vi "NI VeriStand - Get Custom Device Channel Value Table.vi"(8 "error in (no error)":errorcluster, 11 "Channel Ref in":T1 format="%.0x") -> (0 "error out":errorcluster, 1 "Values":dbl[](array[numeric]), 2 "Names":string[](array[string]), 3 "Channel Ref out":T1=18446744073709551615 format="%.0x")   [LabVIEW 2020, in "Custom Device API.lvlib"]
uses:
  <vilib>/NI VeriStand/Custom Device API/Custom Device API.lvlib
  <vilib>/NI VeriStand/Custom Device API/Custom Device Item Ref.ctl
  46f13d71-0576-4d04-b334-0d328d6cd7fa.vi
  <vilib>/NI VeriStand/Custom Device API/Custom Device Offline Path.vi
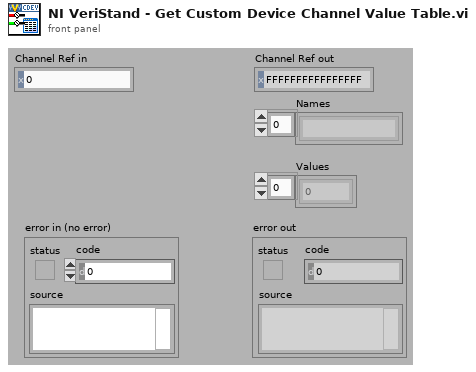
[diagram p1: front panel]
types:
  T1 = typedef "Custom Device API.lvlib/Custom Device Item Ref.ctl" = u64
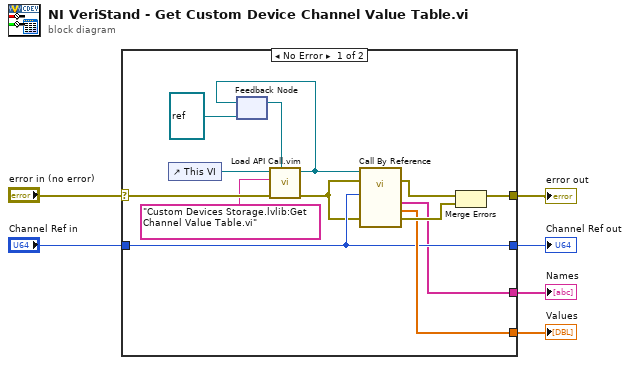
[diagram p0: block diagram]
diagram:
  n1 = case shown="No Error" "error in (no error)" {
    selector: "error in (no error)" -> [w12 w21]
    tunnel: [w17 w21] -> w6
    tunnel: "Channel Ref in" -> [w16 w20]
    tunnel: [w16 w20] -> w4
    tunnel: [w15 _] -> w2
    tunnel: [w18 _] -> w1
    frame No Error {
      n2 = control-ref of="This VI"() -> (w13:refnum<vi>)
      n3 = feedback #1(refnum<vi> refnum ("type specifier VI Refnum (for type only)")) -> (w14:refnum<vi>)
      n4 = call "Load API Call.vim"("VI reference in"=w14, "error in (no error)"=w12, "VI qualified name"="Custom Devices Storage.lvlib:Get Channel Value Table.vi", "Caller VI ref"=w13) -> ("error out"=w11:errorcluster, "VI reference"=w10:refnum<vi>)  [unwired: 6 in]
      n5 = feedback-in #1(w10) -> ()
      n6 = call-by-ref "?"(reference=w10, error in=w11, 8:"error in (no error)"=w11, "Channel Ref in"=w16) -> (error out=w7:errorcluster, 0:"error out"=w19:errorcluster, "Values"=w18:dbl[], "Names"=w15:string[])  [unwired: 6 in, 2 out]
      n7 = Merge Errors(w7, w19) -> (w17:errorcluster)
    }
    frame Error {
    }
  }
  "error out" <- w6
  "Channel Ref out" <- w4
  "Names" <- w2
  "Values" <- w1
